vi "List Instances.vi"(8 "error in (no error)":errorcluster) -> (0 "error out":errorcluster, 2 "First Module ID":i32, 3 "Module IDs":i32[](array[numeric]), 4 "First?":bool[](array[boolean]), 5 "Instances Names":string[](array[string]))   [LabVIEW 2015, in "Chat Window.lvlib" / "Clone Registration.lvlib"]
doc: "Retrieve information on all cloneable modules stored in the registry.\n_____\nBased on Delacor QMH Project Template 4.2.1.64."
uses:
  Clone Registration.lvlib
  Action--enum.ctl
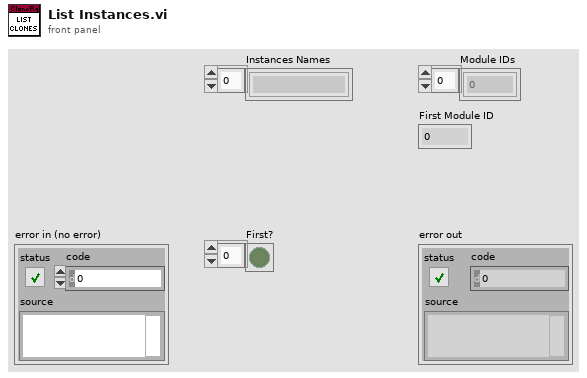
[diagram p1: front panel]
types:
  T1 = typedef "Chat Window.lvlib/Clone Registration.lvlib/Action--enum.ctl" = enum16{"Init", "Add Instance", "Remove Instance", "List Instances", "Is First?"}
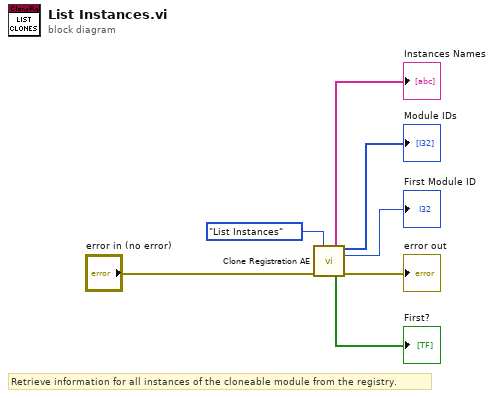
[diagram p0: block diagram]
diagram:
  # "Retrieve information for all instances of the cloneable module from the registry."
  n1 = call "Clone Registration AE.vi"("Action"=Action--enum."List Instances", "error in (no error)"="error in (no error)") -> ("Instances Names"=→"Instances Names":string[], "Module IDs"=→"Module IDs":i32[], "First Module ID"=→"First Module ID":i32, "First? (all)"=→"First?":bool[], "error out"=→"error out":errorcluster)  [unwired: 6 in, 3 out]
